vi "BRAM_ReadDrawPlayfield.vi"(0 "Player IN":u8, 3 "Address":i16) -> (14 "Player OUT":u8, 17 "Data":fxp<+,3,3>)   [LabVIEW 2018]
uses:
  <vilib>/rvi/Memory/Memory_Emulation/nirvimemoryFastEmulation.vi
  <vilib>/rvi/Memory/Memory_Emulation/nirvimemoryEmulation.vi
  <vilib>/rvi/Emulation/niFpgaEmulationIsFPGAContextNoSignature.vi
  <vilib>/rvi/DataTransferAndStorage/Container/Common/niFpgaContainerGetUniqueNameForEmu.vi
  <vilib>/rvi/Emulation/niFpgaProcessEmulError.vi
  <vilib>/rvi/Emulation/niFpgaSctlEmulationGetInTimedLoop.vi
  <vilib>/rvi/errors/nirviReportUnexpectedCaseInternalError (U32).vi
  <vilib>/rvi/DataTransferAndStorage/Container/XNode/niFpgaContainer.xnode
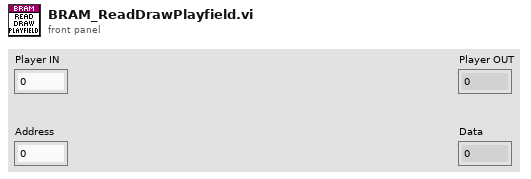
[diagram p1: front panel]
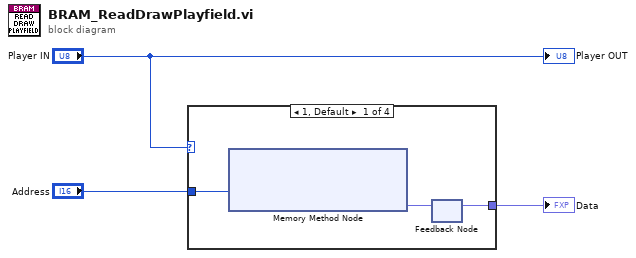
[diagram p0: block diagram]
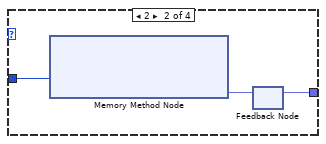
[diagram p2: hidden frame]
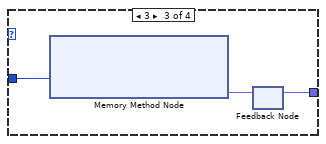
[diagram p3: hidden frame]
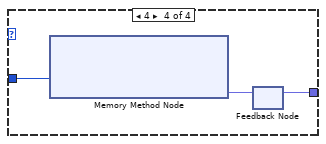
[diagram p4: hidden frame]
diagram:
  n1 = case shown="1, Default" "Player IN" {
    tunnel: [w6 w9 w12 w15] -> w3
    tunnel: "Address" -> [w4 w7 w10 w13]
    frame 1, Default {
      n2 = xnode ("Memory Method Node")("Address"=w4) -> ("Data"=w5:fxp<+,3,3>)  [unwired: 1 in, 1 out]
      n3 = feedback #1() -> (w6:fxp<+,3,3>)  [unwired: 1 in]
      n4 = feedback-in #1(w5) -> ()
    }
    frame 2 {
      n5 = xnode ("Memory Method Node")("Address"=w7) -> ("Data"=w8:fxp<+,3,3>)  [unwired: 1 in, 1 out]
      n6 = feedback #2() -> (w9:fxp<+,3,3>)  [unwired: 1 in]
      n7 = feedback-in #2(w8) -> ()
    }
    frame 3 {
      n8 = xnode ("Memory Method Node")("Address"=w10) -> ("Data"=w11:fxp<+,3,3>)  [unwired: 1 in, 1 out]
      n9 = feedback #3() -> (w12:fxp<+,3,3>)  [unwired: 1 in]
      n10 = feedback-in #3(w11) -> ()
    }
    frame 4 {
      n11 = xnode ("Memory Method Node")("Address"=w13) -> ("Data"=w14:fxp<+,3,3>)  [unwired: 1 in, 1 out]
      n12 = feedback #4() -> (w15:fxp<+,3,3>)  [unwired: 1 in]
      n13 = feedback-in #4(w14) -> ()
    }
  }
  "Data" <- w3
  "Player OUT" <- "Player IN"
